vi "Flatten Buffer Configuration.vi"(11 "Buffer Configuration":T1) -> (3 "Flattened Configuration":u8[](array[numeric]) format="%.0x")   [LabVIEW 2021, in "CIF_CIPC_Chn.lvclass"]
uses:
  CIF_CIPC_Chn.lvclass
  Typedef/Buffer Configuration Data.ctl
  <vilib>/CIF Foundation/CIF CIPC/TypeDefs/Backpressure References.ctl
  CIF_CIPC_Chn.lvclass/CIF_CIPC_Chn.ctl
  <vilib>/CIF Foundation/CIF Utilities/DataTypes/DataTypes_CIF_U.lvlib
  <vilib>/CIF Foundation/CIF CIPC/CIF_NI_CIPC.lvlib
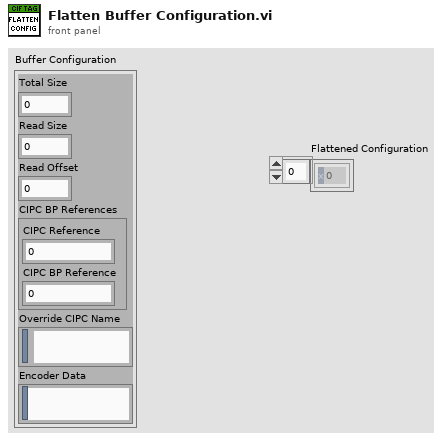
[diagram p1: front panel]
types:
  T1 = typedef "CIF_CIPC_Chn.lvclass/Buffer Configuration Data.ctl" = cluster{"Total Size":u32, "Read Size":u32, "Read Offset":u32, "CIPC BP References":T2, "Override CIPC Name":string, "Encoder Data":string}
  T2 = typedef "CIF_NI_CIPC.lvlib/Backpressure References.ctl" = cluster{"CIPC Reference":u64, "CIPC BP Reference":u64}
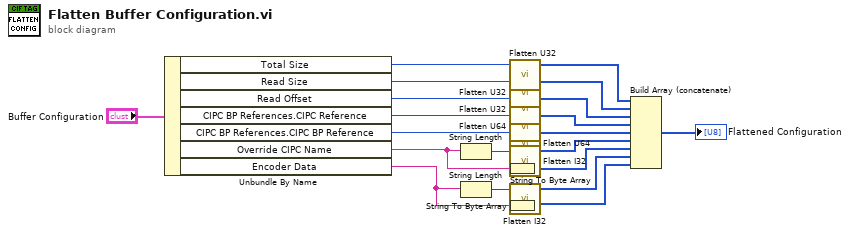
[diagram p0: block diagram]
diagram:
  n1 = Unbundle By Name("Buffer Configuration") -> ("Total Size"=w19:u32, "Read Size"=w17:u32, "Read Offset"=w18:u32, "CIPC BP References.CIPC Reference"=w3:u64, "CIPC BP References.CIPC BP Reference"=w4:u64, "Override CIPC Name"=w10:string, "Encoder Data"=w7:string)
  n2 = String Length(string=w10) -> (length=w12:i32)
  n3 = String Length(string=w7) -> (length=w8:i32)
  n4 = String To Byte Array(string=w10) -> (unsigned byte array=w9:u8[])
  n5 = String To Byte Array(string=w7) -> (unsigned byte array=w5:u8[])
  n6 = call <vilib>:"Flatten U32.vi"("U32"=w19) -> ("Flat Data"=w16:u8[])  [unwired: 4 in]
  n7 = call <vilib>:"Flatten U32.vi"("U32"=w17) -> ("Flat Data"=w15:u8[])  [unwired: 4 in]
  n8 = call <vilib>:"Flatten U32.vi"("U32"=w18) -> ("Flat Data"=w14:u8[])  [unwired: 4 in]
  n9 = call <vilib>:"Flatten U64.vi"("U64"=w3) -> ("Flat Data"=w1:u8[])  [unwired: 4 in]
  n10 = call <vilib>:"Flatten U64.vi"("U64"=w4) -> ("Flat Data"=w2:u8[])  [unwired: 4 in]
  n11 = call <vilib>:"Flatten I32.vi"("I32"=w12) -> ("Flat Data"=w11:u8[])  [unwired: 4 in]
  n12 = call <vilib>:"Flatten I32.vi"("I32"=w8) -> ("Flat Data"=w6:u8[])  [unwired: 4 in]
  n13 = Build Array (concatenate)(w16, w15, w14, w1, w2, w11, w9, w6, w5) -> (→"Flattened Configuration":u8[])
